vi "motion_kd.vi"() -> ()   [LabVIEW 2012]
uses:
  <vilib>/Motion/FlexMotion/CustomControls/CustomControls.llb/Axis # (8 axes).flx
  <vilib>/Platform/TimedLoop/XDataNode/timing_clust.ctl
  <vilib>/Platform/TimedLoop/XDataNode/nitl_modes.ctl
  <vilib>/Platform/TimedLoop/XDataNode/wakeup.ctl
  <vilib>/Motion/FlexMotion/FunctionsVIs/StartStopMotion.llb/Stop Motion (8 axes).flx
  <vilib>/platform/TimedLoop/XDataNode/XDataNode.xnode
  <vilib>/Platform/TimedLoop/XDataNode/XDNodeRunTimeDep.lvlib
panel:
  in  "SAVP":i32=4 min=1
  in  "MAV":i32=4 min=1
  in  "stop 2":bool
  out "XY Graph":cluster{"Array out":dbl[], "Array out":dbl[]}(graph)
  out "Waveform Chart 2":i64(graph)=61900
  out "Waveform Chart":i32(graph)=13718
  out "Current position":T1={"Axis 1"=0, "Axis 2"=13718.0, "Axis 3"=0, "Axis 4"=0}
  in  "start":bool
  in  "Motion Parameters":T3={"Motion Board ID"=1, "Axis parameters in"=[{"Axis type"=0, " Velocity (rpm)"=4.0, " Acceln (rps\\s)"=1.0, " Deceln (rps\\s)"=1.0, "Enc Counts/Rev"=2880, "Kp"=30, "Kd"=800, "Td"=2}, {"Axis type"=0, " Velocity (rpm)"=200.0, " Acceln (rps\\s)"=0.05, " Deceln (rps\\s)"=0.5, "Enc Counts/Rev"=2880, "Kp"=100, "Kd"=1000, "Td"=2}, {"Axis type"=0, " Velocity (rpm)"=4000.0, " Acceln (rps\\s)"=1000.0, " Deceln (rps\\s)"=1000.0, "Enc Counts/Rev"=8000, "Kp"=60, "Kd"=700, "Td"=5}, {"Axis type"=0, " Velocity (rpm)"=4000.0, " Acceln (rps\\s)"=1000.0, " Deceln (rps\\s)"=1000.0, "Enc Counts/Rev"=8000, "Kp"=60, "Kd"=700, "Td"=5}], "Axis status"={"Axis 1"=FALSE, "Axis 2"=TRUE, "Axis 3"=FALSE, "Axis 4"=FALSE, "Axis 5"=FALSE, "Axis 6"=FALSE, "Axis 7"=FALSE, "Axis 8"=FALSE}, "Current position"={"Axis 1"=0.0, "Axis 2"=0.0, "Axis 3"=0.0, "Axis 4"=0.0}} {"Axis parameters in"."Axis type" items=["Free axis", "Master axis", "Slave axis"]; "Axis parameters in"."Enc Counts/Rev" min=1; "Axis parameters in"."Deceln (rps\\s)" max=2097152.0 step=0.1 format="%.2f"; "Axis parameters in"."Acceln (rps\\s)" min=0.0 max=2097152.0 format="%.2f"; "Axis parameters in"."Velocity (rpm)" min=-536870912.0 max=536870912.0 step=1.0 format="%.2f"; "Axis parameters in"."Td" max=63; "Axis parameters in"."Kd" max=32767; "Axis parameters in"."Kp" max=32767; "Motion Board ID" min=1 max=32 step=1}
  out "error out":errorcluster
  in  "stop":bool
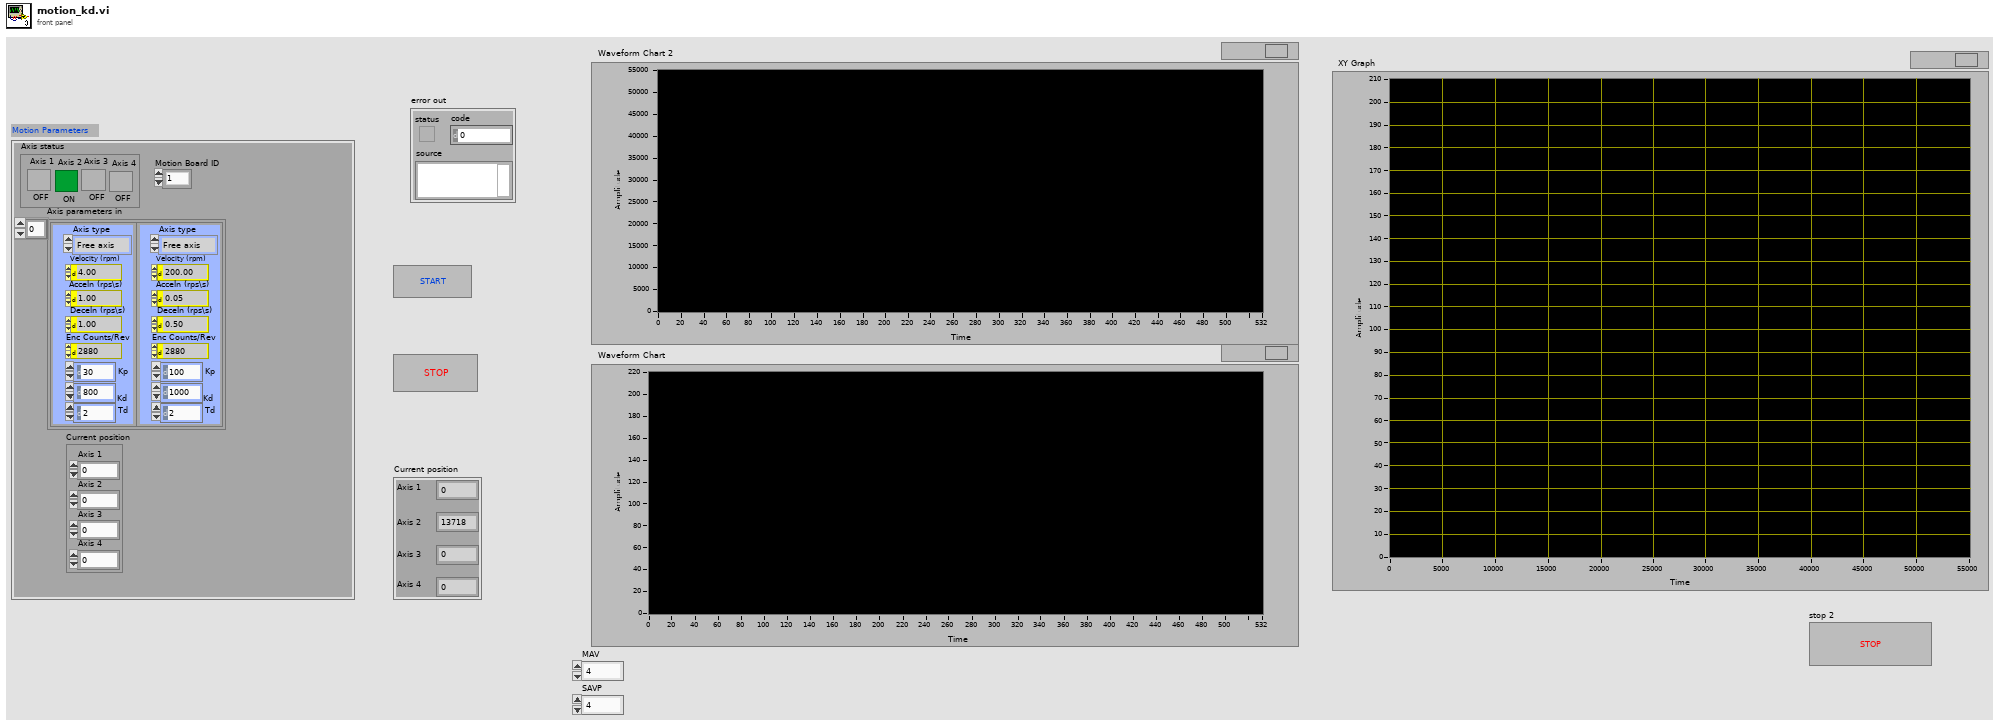
[diagram p1: front panel]
types:
  T1 = cluster{"Axis 1":i32, "Axis 2":dbl, "Axis 3":i32, "Axis 4":i32}
  T2 = typedef "Board Id" = u8
  T3 = cluster{"Motion Board ID":T2, "Axis parameters in":cluster{"Axis type":u16, " Velocity (rpm)":dbl, " Acceln (rps\\s)":dbl, " Deceln (rps\\s)":dbl, "Enc Counts/Rev":u16, "Kp":u16, "Kd":u16, "Td":u16}[], "Axis status":cluster{"Axis 1":bool, "Axis 2":bool, "Axis 3":bool, "Axis 4":bool, "Axis 5":bool, "Axis 6":bool, "Axis 7":bool, "Axis 8":bool}, "Current position":cluster{"Axis 1":dbl, "Axis 2":dbl, "Axis 3":dbl, "Axis 4":dbl}}
  T4 = typedef "Axis # (8 axes).flx" = cluster{"1":bool, "2":bool, "3":bool, "4":bool, "5":bool, "6":bool, "7":bool, "8":bool}
  T5 = cluster{"Motion Board ID":T2, "Axis parameters in":cluster{"Axis type":u16, "Velocity (rpm)":dbl, "Acceln (rps\\s)":dbl, "Deceln (rps\\s)":dbl, "Enc Counts/Rev":u16, "Kp":u16, "Kd":u16, "Td":u16}[], "Axis status":cluster{"Axis 1":bool, "Axis 2":bool, "Axis 3":bool, "Axis 4":bool, "Axis 5":bool, "Axis 6":bool, "Axis 7":bool, "Axis 8":bool}, "Current position":cluster{"Axis 1":dbl, "Axis 2":dbl, "Axis 3":dbl, "Axis 4":dbl}}
  T6 = typedef "XDNodeRunTimeDep.lvlib/timing_clust.ctl" = cluster{"Expected End [f-1]":u64, "Actual End [f-1]":u64, "Finished Late? [f-1]":bool, "Expected End [i-1]":u64, "Actual End [i-1]":u64, "Finished Late? [i-1]":bool, "Expected Start [i]":u64, "Actual Start [i]":u64, "Expected Start [f]":u64, "Actual Start [f]":u64, "Source Name":string, "Structure Name":string, "Period":i64, "Deadline":i64, "Offset":i64, "Start":i64, "Priority":i32, "Timeout":i32, "Mode":T7, "Wakeup Reason":T8, "Error":errorcluster, "Source Type":string, "Secondary Source Type":string, "Global End Time":u64, "Global Start Time":u64, "Frame Duration":u64, "Iteration Duration":u64, "Assigned CPU":i32, "I/O Scan Engine Mode":u32}
  T7 = typedef "XDNodeRunTimeDep.lvlib/nitl_modes.ctl" = enum32{"No Change", "Process missed periods, maintain original phase", "Discard missed periods, maintain original phase", "Process missed periods, ignore original phase", "Discard missed periods, ignore original phase"}
  T8 = typedef "XDNodeRunTimeDep.lvlib/wakeup.ctl" = enum32{"Normal", "Aborted", "Asynchronous wakeup", "Timing source error", "Timed loop error", "Timeout"}
  T9 = cluster{"Axis 1":i32, "Axis 2":i32, "Axis 3":i32, "Axis 4":i32}
  T10 = cluster{"Axis 1":bool, "Axis 2":bool, "Axis 3":bool, "Axis 4":bool, "Axis 5":bool, "Axis 6":bool, "Axis 7":bool, "Axis 8":bool}
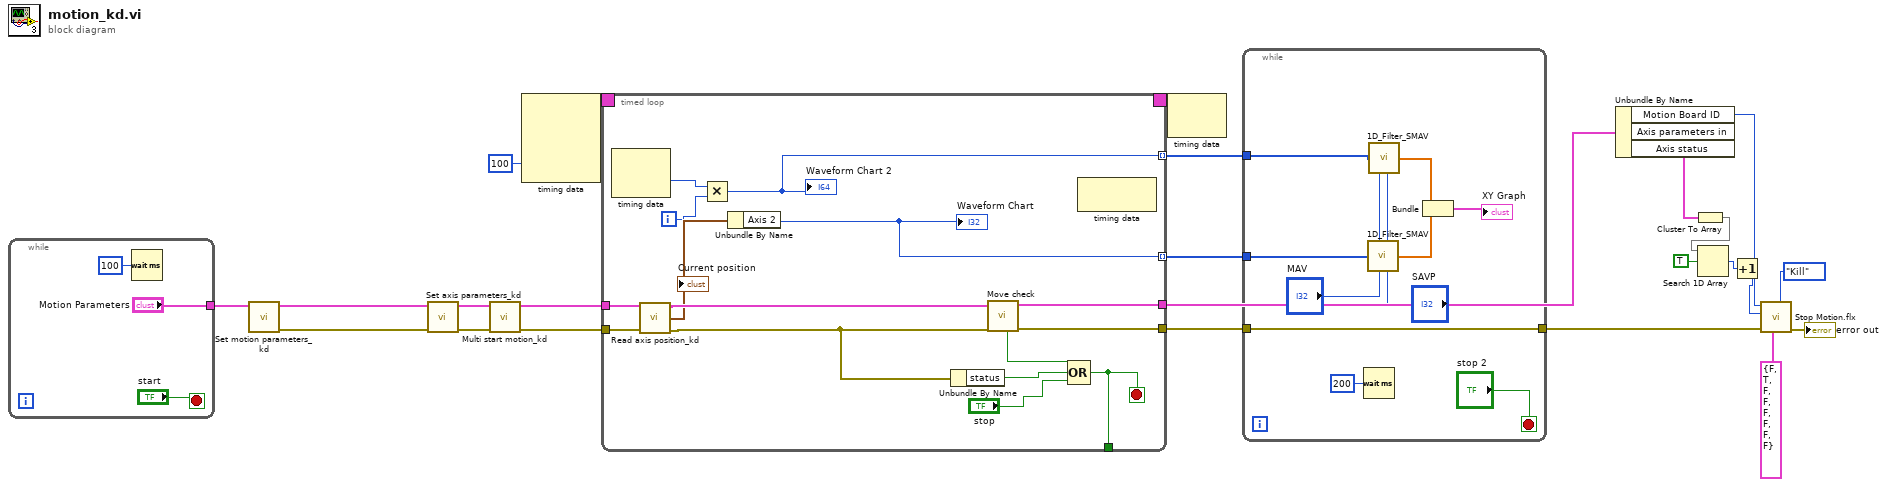
[diagram p0: block diagram]
diagram:
  n1 = while {
    tunnel: ["Motion Parameters"] -> w22
    stop <- "start" stop-if-true
    n2 = Wait (ms)(milliseconds to wait=u32 100) -> ()  [unwired: 1 out]
  }
  n3 = call "Set motion parameters_kd.vi"("Motion Parameters"=w22) -> ("error out"=w24:errorcluster, "Motion Para out"=w23:T3)  [unwired: 9 in]
  n4 = call "Set axis parameters_kd.vi"("error in"=w24, "Motion Parameters"=w23) -> ("error out"=w9:errorcluster, "Motion para out"=w8:T5)  [unwired: 7 in]
  n5 = call "Multi start motion_kd.vi"("error in"=w9, "Motion Parameters"=w8) -> ("error out"=w6:errorcluster, "Motion Para out"=w7:T3)  [unwired: 6 in]
  n6 = node-c288(i64 100 ("Period")) -> (w11:T6)  [unwired: 3 in]
  n7 = timed-loop {
    tunnel: w7 -> [w42]
    tunnel: w6 -> [w41]
    tunnel: [w40] -> w2
    tunnel: [w39] -> w18
    tunnel: [w33] -> _
    timing: w11 -> [_]
    timing-out: [_] -> w10
    tunnel: [w29] -> w4 mode=indexing
    tunnel: [w28] -> w3 mode=indexing
    i -> [w30]
    stop <- w33 stop-if-true
    n8 = node-c288() -> (w31:i64)  [unwired: 1 in, 1 out]
    n9 = call "Read axis position_kd.vi"("error in"=w41, "Motion Parameters"=w42) -> ("error out"=w37:errorcluster, "Motion Para out"=w38:T3, "Current position"=w32:T9)  [unwired: 5 in]
    "Current position" <- w32
    n10 = Multiply(x=w31, y=w30) -> (x*y=w29:i64)
    "Waveform Chart 2" <- w29
    n11 = Unbundle By Name(w32) -> ("Axis 2"=w28:i32)
    "Waveform Chart" <- w28
    n12 = Unbundle By Name(w37) -> ("status"=w35:bool)
    n13 = call "Move check.vi"("error in"=w37, "Motion Parameters"=w38) -> ("error out"=w40:errorcluster, "Motion Para out"=w39:T3, "Move Complete"=w36:bool)  [unwired: 5 in]
    n14 = Compound Arithmetic op=OR(w36, w35, "stop") -> (w33:bool)
    n15 = node-c288() -> ()  [unwired: 1 in, 1 out]
  }
  n16 = node-c288(w10) -> ()  [unwired: 1 out]
  n17 = while {
    tunnel: w4 -> [w54]
    tunnel: w3 -> [w52]
    tunnel: w2 -> [w50]
    tunnel: [w50] -> w1
    stop <- "stop 2" stop-if-true
    n18 = Wait (ms)(milliseconds to wait=u32 200) -> ()  [unwired: 1 out]
    n19 = call "1D_Filter_SMAV.vi"("Array in"=w52, "MAV"="MAV", "SAVP"="SAVP") -> ("Array out"=w51:dbl[])
    n20 = call "1D_Filter_SMAV.vi"("Array in"=w54, "MAV"="MAV", "SAVP"="SAVP") -> ("Array out"=w53:dbl[])
    n21 = Bundle("Array out"=w53, "Array out"=w51) -> (→"XY Graph":cluster{"Array out":dbl[], "Array out":dbl[]})  [unwired: 1 in]
  }
  n22 = Unbundle By Name(w18) -> ("Motion Board ID"=w17:T2, "Axis status"=w16:T10)  [unwired: 1 out]
  n23 = Cluster To Array(cluster=w16) -> (array=w15:bool[])
  n24 = Search 1D Array(1D array=w15, element=TRUE) -> (index of element=w13:i32)  [unwired: 1 in]
  n25 = Increment(x=w13) -> (x+1=w12:i32)
  n26 = call-poly <vilib>:"Stop Motion.flx"("Stop Type (Decel)"=enum16{"Decelerate", "Halt", "Kill"}."Kill", "Axis/VS Map (Disabled)"=T4 {"1"=FALSE, "2"=TRUE, "3"=FALSE, "4"=FALSE, "5"=FALSE, "6"=FALSE, "7"=FALSE, "8"=FALSE}, "error in (no error)"=w1, "Axis or Vector Space"=w12, "Board ID"=w17) -> ("error out"=→"error out":errorcluster)  [unwired: 2 in, 2 out]
